vi "create index groupings.vi"(8 "error in":errorcluster, 11 "data dictionary":refnum<class "data dictionary.lvclass">) -> (0 "error out":errorcluster, 2 "indices":T1[](array[typedef]))   [LabVIEW 2013, in "CVT runtime.lvclass"]
uses:
  CVT runtime.lvclass
  <vilib>/NI/Current Value Table/Type Defs/Typed Index Set.ctl
  <vilib>/NI/Current Value Table/Type Defs/Data Types.ctl
  <vilib>/NI/Tag Bus/dictionary/data dictionary.lvclass
  <vilib>/NI/Current Value Table/Type Defs/Single Tag.ctl
  <vilib>/NI/Current Value Table/Type Defs/File Format.ctl
  <vilib>/NI/Current Value Table/Type Defs/Tag Grouping set.ctl
  <vilib>/NI/Current Value Table/Errors/Generate Error.vi
  <vilib>/NI/Current Value Table/FGVs/Tag Memory.vi
  <vilib>/NI/Current Value Table/Current Value Table.lvlib
  <vilib>/NI/Tag Bus/tag/tag descriptor.lvclass
  configuration/CVT configuration.lvclass
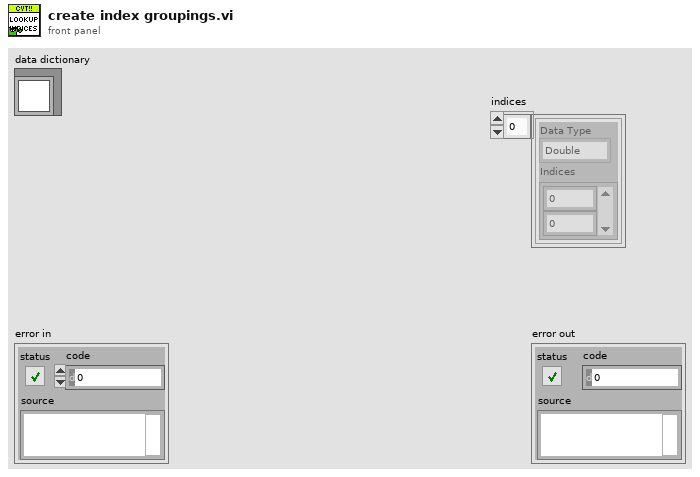
[diagram p1: front panel]
types:
  T1 = typedef "Current Value Table.lvlib/Typed Index Set.ctl" = cluster{"Data Type":T2, "Indices":i32[]}
  T2 = typedef "Current Value Table.lvlib/Data Types.ctl" = enum16{"Double", "Single", "I64", "I32", "I16", "I8", "U64", "U32", "U16", "U8", "String", "Boolean", "Array of U8", "Array of U16", "Array of U32", "Array of U64", "Array of I64", "Array of I32", "Array of I16", "Array of I8", "Array of Double", "Array of Single", "Array of Boolean", "Array of String"}
  T3 = typedef "tag bus.lvlib/data dictionary.lvclass/full data dictionary.ctl" = cluster{"Double":string[], "Single":string[], "I64":string[], "I32":string[], "I16":string[], "I8":string[], "U64":string[], "U32":string[], "U16":string[], "U8":string[], "Boolean":string[], "String":string[], "Array of Double":string[], "Array of Single":string[], "Array of I64":string[], "Array of I32":string[], "Array of I16":string[], "Array of I8":string[], "Array of U64":string[], "Array of U32":string[], "Array of U16":string[], "Array of U8":string[], "Array of Boolean":string[], "Array of String":string[]}
  T4 = typedef "Current Value Table.lvlib/File Format.ctl" = cluster{"Tags":T5[], "Group Listings":T6[]}
  T5 = typedef "Current Value Table.lvlib/Single Tag.ctl" = cluster{"Data Type":T2, "Name":string, "Value":string, "Description":string}
  T6 = typedef "Current Value Table.lvlib/Tag Grouping set.ctl" = cluster{"Group":string, "Tag Names":string[]}
  T7 = typedef "tag bus.lvlib/tag descriptor.lvclass/Data Type.ctl" = enum16{"Double", "Single", "I64", "I32", "I16", "I8", "U64", "U32", "U16", "U8", "Boolean", "String", "Array of Double", "Array of Single", "Array of I64", "Array of I32", "Array of I16", "Array of I8", "Array of U64", "Array of U32", "Array of U16", "Array of U8", "Array of Boolean", "Array of String"}
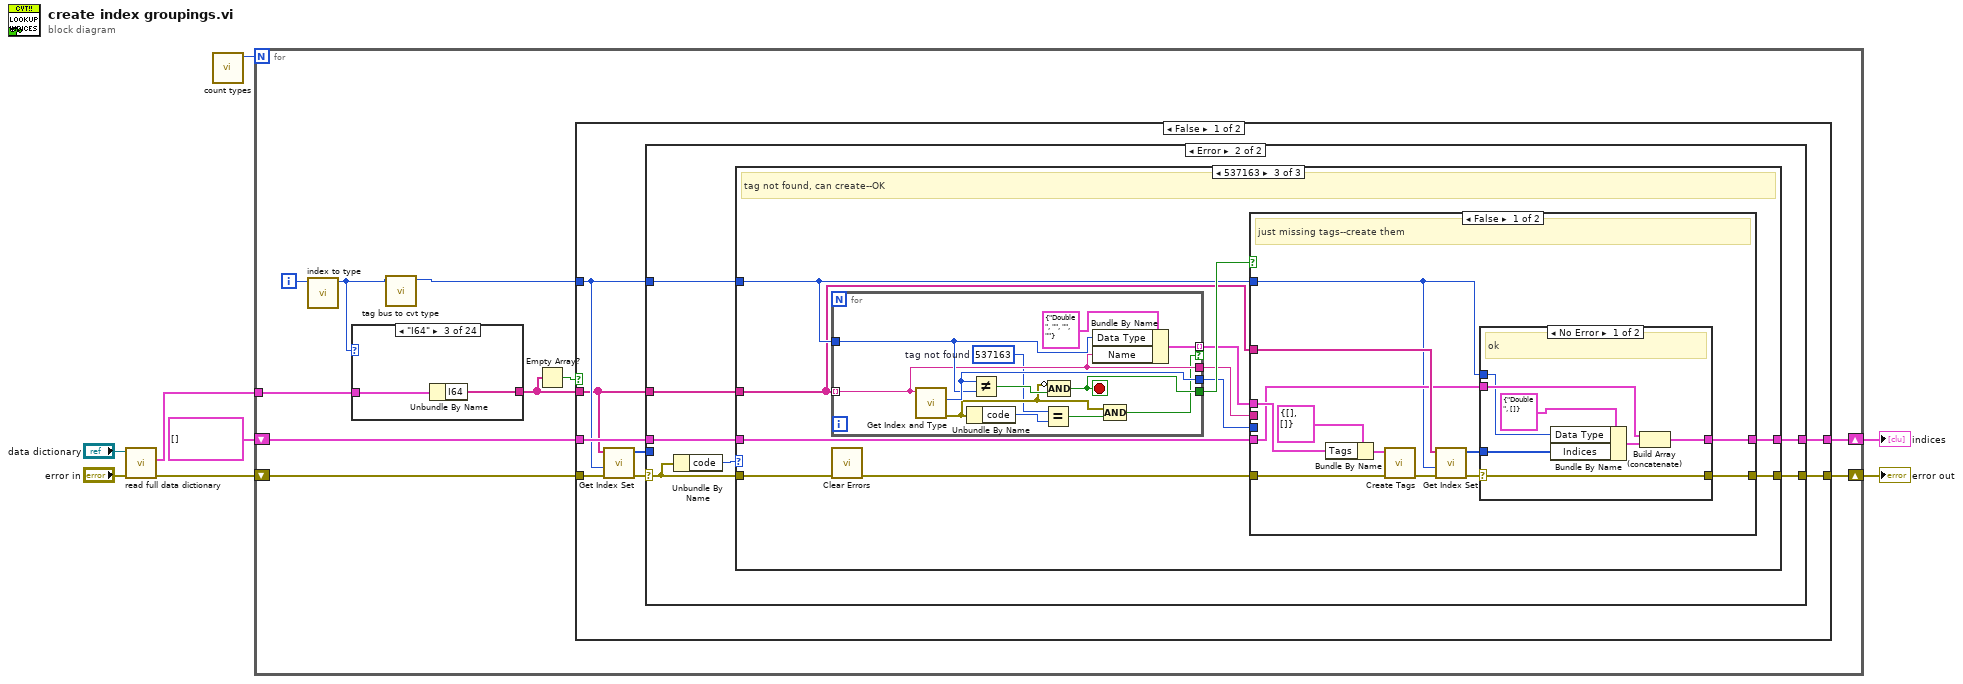
[diagram p0: block diagram]
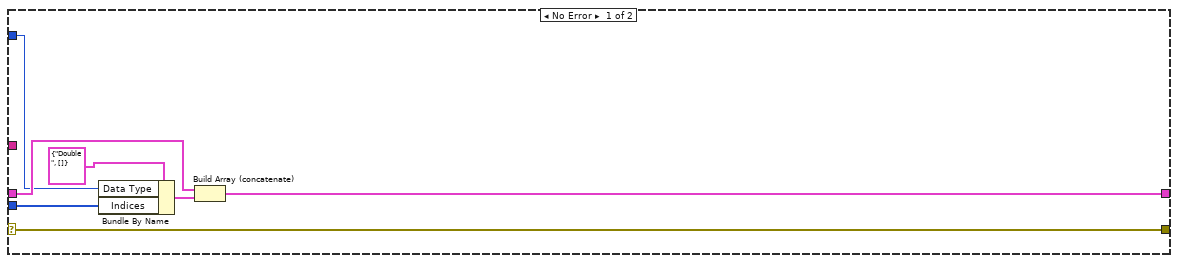
[diagram p2: hidden frame]
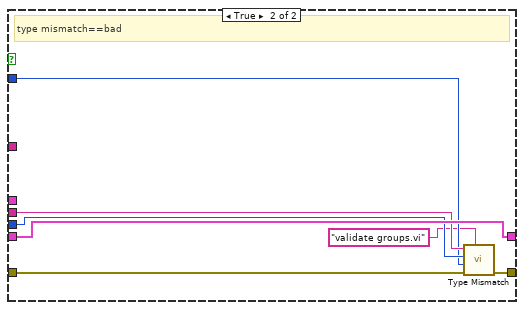
[diagram p6: hidden frame]
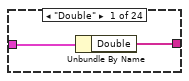
[diagram p8: hidden frame]
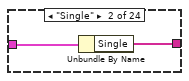
[diagram p9: hidden frame]
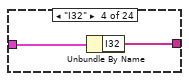
[diagram p10: hidden frame]
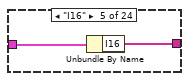
[diagram p11: hidden frame]
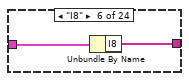
[diagram p12: hidden frame]
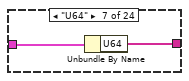
[diagram p13: hidden frame]
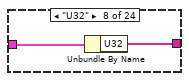
[diagram p14: hidden frame]
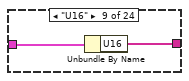
[diagram p15: hidden frame]
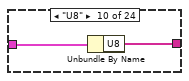
[diagram p16: hidden frame]
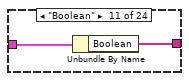
[diagram p17: hidden frame]
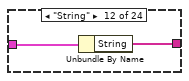
[diagram p18: hidden frame]
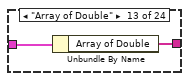
[diagram p19: hidden frame]
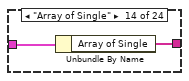
[diagram p20: hidden frame]
diagram:
  n1 = call <vilib>:"read full data dictionary.vi"("error in"="error in", "data dictionary in"="data dictionary") -> ("error out"=w3:errorcluster, "dictionary"=w1:T3)  [unwired: 7 in, 1 out]
  n2 = call <vilib>:"count types.vi"() -> ("type count"=w8:i32)  [unwired: 11 in]
  n3 = for {
    N: w8 -> [_]
    shift-right: [w18] -> w6
    shift-left: T1[] [] -> [w17]
    shift-right: [w15] -> w7
    shift-left: w3 -> [w16]
    tunnel: w1 -> [w13]
    i -> [w14]
    n4 = call <vilib>:"index to type.vi"("I32"=w14) -> ("type"=w10:T7)  [unwired: 10 in]
    n5 = case shown="\"I64\"" w10 {
      tunnel: w13 -> [w99 w101 w103 w105 w107 w109 w111 w113 w115 w117 w119 w121 w123 w125 w127 w129 w131 w133 w135 w137 w139 w141 w143 w145]
      tunnel: [w98 w100 w102 w104 w106 w108 w110 w112 w114 w116 w118 w120 w122 w124 w126 w128 w130 w132 w134 w136 w138 w140 w142 w144] -> w12
      frame "Double" {
        n6 = Unbundle By Name(w99) -> ("Double"=w98:string[])
      }
      frame "Single" {
        n7 = Unbundle By Name(w101) -> ("Single"=w100:string[])
      }
      frame "I64" {
        n8 = Unbundle By Name(w103) -> ("I64"=w102:string[])
      }
      frame "I32" {
        n9 = Unbundle By Name(w105) -> ("I32"=w104:string[])
      }
      frame "I16" {
        n10 = Unbundle By Name(w107) -> ("I16"=w106:string[])
      }
      frame "I8" {
        n11 = Unbundle By Name(w109) -> ("I8"=w108:string[])
      }
      frame "U64" {
        n12 = Unbundle By Name(w111) -> ("U64"=w110:string[])
      }
      frame "U32" {
        n13 = Unbundle By Name(w113) -> ("U32"=w112:string[])
      }
      frame "U16" {
        n14 = Unbundle By Name(w115) -> ("U16"=w114:string[])
      }
      frame "U8" {
        n15 = Unbundle By Name(w117) -> ("U8"=w116:string[])
      }
      frame "Boolean" {
        n16 = Unbundle By Name(w119) -> ("Boolean"=w118:string[])
      }
      frame "String" {
        n17 = Unbundle By Name(w121) -> ("String"=w120:string[])
      }
      frame "Array of Double" {
        n18 = Unbundle By Name(w123) -> ("Array of Double"=w122:string[])
      }
      frame "Array of Single" {
        n19 = Unbundle By Name(w125) -> ("Array of Single"=w124:string[])
      }
      frame "Array of I64" {
        n20 = Unbundle By Name(w127) -> ("Array of I64"=w126:string[])
      }
      frame "Array of I32" {
        n21 = Unbundle By Name(w129) -> ("Array of I32"=w128:string[])
      }
      frame "Array of I16" {
        n22 = Unbundle By Name(w131) -> ("Array of I16"=w130:string[])
      }
      frame "Array of I8" {
        n23 = Unbundle By Name(w133) -> ("Array of I8"=w132:string[])
      }
      frame "Array of U64" {
        n24 = Unbundle By Name(w135) -> ("Array of U64"=w134:string[])
      }
      frame "Array of U32" {
        n25 = Unbundle By Name(w137) -> ("Array of U32"=w136:string[])
      }
      frame "Array of U16" {
        n26 = Unbundle By Name(w139) -> ("Array of U16"=w138:string[])
      }
      frame "Array of U8" {
        n27 = Unbundle By Name(w141) -> ("Array of U8"=w140:string[])
      }
      frame "Array of Boolean" {
        n28 = Unbundle By Name(w143) -> ("Array of Boolean"=w142:string[])
      }
      frame "Array of String" {
        n29 = Unbundle By Name(w145) -> ("Array of String"=w144:string[])
      }
    }
    n30 = call "tag bus to cvt type.vi"("Data Type"=w10) -> ("cvt type"=w9:T2)  [unwired: 10 in]
    n31 = Empty Array?(array=w12) -> (empty?=w11:bool)
    n32 = case shown="False" w11 {
      tunnel: [w26 w97] -> w18
      tunnel: w17 -> [w25 w97]
      tunnel: w16 -> [w24 w96]
      tunnel: [w23 w96] -> w15
      tunnel: w9 -> [w20 _]
      tunnel: w12 -> [w19 _]
      frame False {
        n33 = call <vilib>:"Get Index Set.vi"("error in (no error)"=w24, "Expected Type"=w20, "Tag Names"=w19) -> ("error out"=w22:errorcluster, "Tag References"=w21:i32[])  [unwired: 7 in]
        n34 = case shown="Error" w22 {
          selector: w22 -> [w33 w36]
          tunnel: [w33 w37] -> w23
          tunnel: w25 -> [w31 w39]
          tunnel: [w30 w38] -> w26
          tunnel: w20 -> [w28 w34]
          tunnel: w21 -> [w27 _]
          tunnel: w19 -> [_ w35]
          frame No Error {
            n35 = Bundle By Name(cluster=T1 {"Data Type"=enum."Double", "Indices"=[]} ("Index Type Set"), "Data Type"=w28, "Indices"=w27) -> (w29:T1)
            n36 = Build Array (concatenate)(w31, w29) -> (w30:T1[])
          }
          frame Error {
            n37 = Unbundle By Name(w36) -> ("code"=w40:i32)
            n38 = case shown="537163" w40 {
              tunnel: w39 -> [w41 w44 w51]
              tunnel: [w41 w44 w52] -> w38
              tunnel: [w42 w43 w53] -> w37
              tunnel: w36 -> [w42 w43 w55]
              tunnel: w35 -> [_ _ w45]
              tunnel: w34 -> [_ _ w47]
              frame Default {
                # "unk"
              }
              frame 537165 {
                # "tag found but type mismatch"
              }
              frame 537163 {
                # "tag not found, can create--OK"
                n39 = for {
                  tunnel: w45 -> [w89] mode=indexing
                  tunnel: w47 -> [w90]
                  tunnel: [w94] -> w50
                  tunnel: [w89] -> w49
                  tunnel: [w93] -> w48
                  tunnel: [w91] -> w46 mode=indexing if=w84
                  stop <- w94 stop-if-true
                  w85 = 537163  # tag not found
                  n40 = call <vilib>:"Get Index and Type.vi"("Tag"=w89) -> ("error out"=w86:errorcluster, "Type"=w93:T2)  [unwired: 8 in, 1 out]
                  n41 = Unbundle By Name(w86) -> ("code"=w88:i32)
                  n42 = Not Equal?(x=w93, y=w90) -> (x != y?=w95:bool)
                  n43 = Equal?(x=w85, y=w88) -> (x = y?=w87:bool)
                  n44 = Compound Arithmetic op=AND(invert w86, w95) -> (w94:bool)
                  n45 = Bundle By Name(cluster=T5 {"Data Type"=enum."Double", "Name"="", "Value"="", "Description"=""} ("Tag"), "Data Type"=w90, "Name"=w89) -> (w91:T5)
                  n46 = Compound Arithmetic op=AND(w86, w87) -> (w84:bool)
                }
                n47 = call <vilib>:"Clear Errors.vi"("error in (no error)"=w55) -> ("error out"=w54:errorcluster)  [unwired: 6 in]
                n48 = case shown="False" w50 {
                  tunnel: w54 -> [w67 w83]
                  tunnel: [w63 w82] -> w53
                  tunnel: [w58 w81] -> w52
                  tunnel: w51 -> [w59 w81]
                  tunnel: w49 -> [_ w80]
                  tunnel: w48 -> [_ w79]
                  tunnel: w47 -> [w57 w78]
                  tunnel: w46 -> [w64 _]
                  tunnel: w45 -> [w61 _]
                  frame False {
                    # "just missing tags--create them"
                    n49 = Bundle By Name(cluster=T4 {"Tags"=[], "Group Listings"=[]} ("CVT Tags to Create"), "Tags"=w64) -> (w65:T4)
                    n50 = call <vilib>:"Create Tags.vi"("error in (no error)"=w67, "CVT Tags to Create"=w65) -> ("error out"=w62:errorcluster)  [unwired: 9 in]
                    n51 = call <vilib>:"Get Index Set.vi"("error in (no error)"=w62, "Expected Type"=w57, "Tag Names"=w61) -> ("error out"=w60:errorcluster, "Tag References"=w56:i32[])  [unwired: 7 in]
                    n52 = case shown="No Error" w60 {
                      selector: w60 -> [w74 w76]
                      tunnel: [w74 w76] -> w63
                      tunnel: w59 -> [w71 w75]
                      tunnel: [w70 w75] -> w58
                      tunnel: w57 -> [w69 _]
                      tunnel: w56 -> [w68 _]
                      frame No Error {
                        # "ok"
                        n53 = Bundle By Name(cluster=T1 {"Data Type"=enum."Double", "Indices"=[]} ("Index Type Set"), "Data Type"=w69, "Indices"=w68) -> (w72:T1)
                        n54 = Build Array (concatenate)(w71, w72) -> (w70:T1[])
                      }
                      frame Error {
                        # "unk"
                      }
                    }
                  }
                  frame True {
                    # "type mismatch==bad"
                    n55 = call <vilib>:"Type Mismatch.vi"("caller name"="validate groups.vi", "error in (no error)"=w83, "Data Type Requested"=w78, "True Type"=w79, "Tag"=w80) -> ("error out"=w82:errorcluster)  [unwired: 6 in]
                  }
                }
              }
            }
          }
        }
      }
      frame True {
      }
    }
  }
  "error out" <- w7
  "indices" <- w6
